vi "Draw Flattened Pixmap.vi"(8 "image data":T1, 9 "picture":picture) -> (3 "new picture":picture)   [LabVIEW 2011]
doc: "Draws a 1-, 4-, or 8-bit pixmap or a 24-bit RGB pixmap into a picture."
uses:
  imagedata.ctl
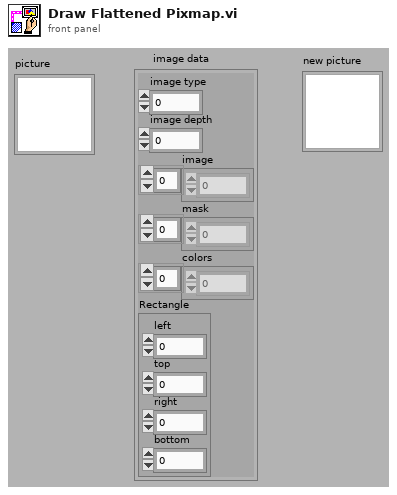
[diagram p1: front panel]
types:
  T1 = typedef "imagedata.ctl" = cluster{"image type":i32, "image depth":i32, "image":u8[], "mask":u8[], "colors":u32[], "Rectangle":cluster{"left":i16, "top":i16, "right":i16, "bottom":i16}}
  T2 = cluster{"left":i16, "top":i16, "right":i16, "bottom":i16}
  T3 = cluster{"top":i16, "left":i16, "bottom":i16, "right":i16}
  T4 = cluster{"default foreground":u32, "default background":u32}
  T5 = cluster{"opcode-Copy Pixmap":i16, i32, i32, cluster{"top":i16, "left":i16, "bottom":i16, "right":i16}, i16, cluster{"default foreground":u32, "default background":u32}}
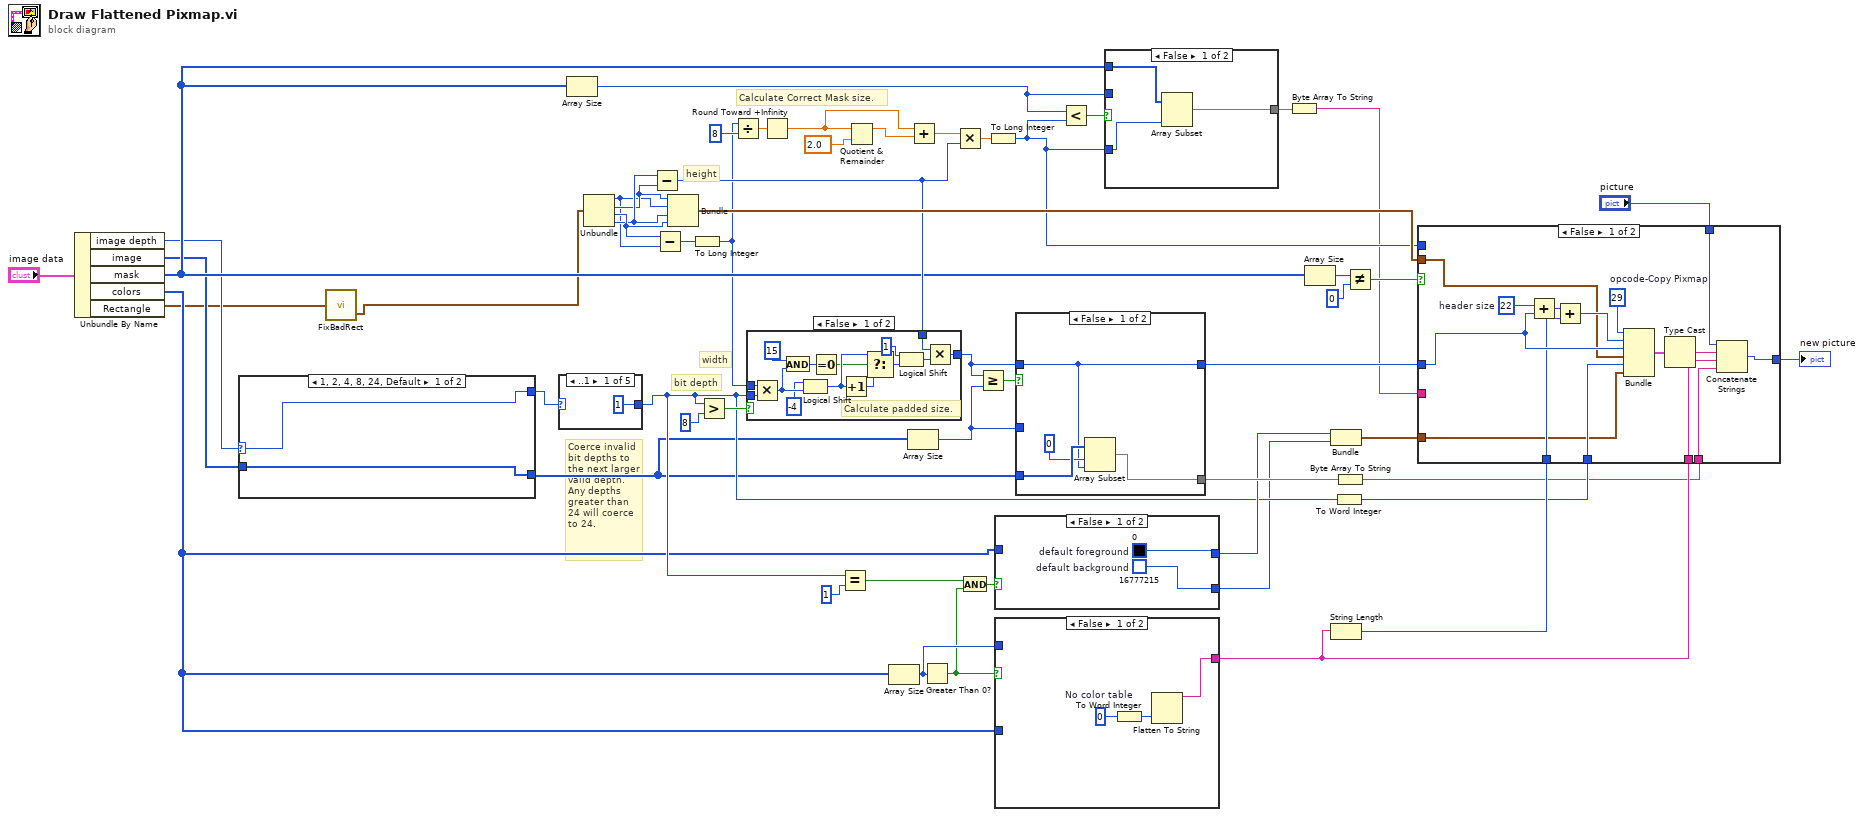
[diagram p0: block diagram]
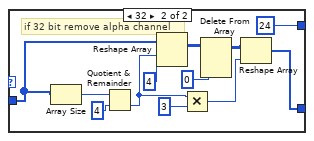
[diagram p2: hidden frame]
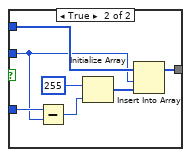
[diagram p3: hidden frame]
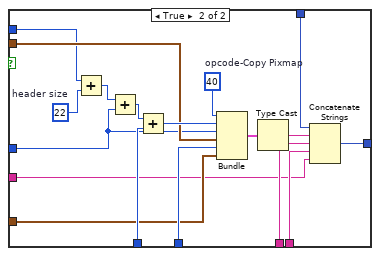
[diagram p4: hidden frame]
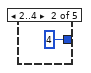
[diagram p5: hidden frame]
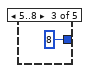
[diagram p6: hidden frame]
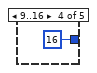
[diagram p7: hidden frame]
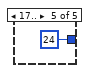
[diagram p8: hidden frame]
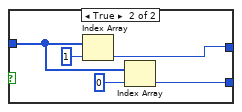
[diagram p9: hidden frame]
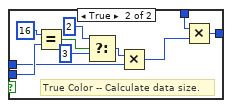
[diagram p10: hidden frame]
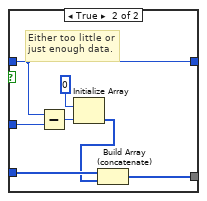
[diagram p11: hidden frame]
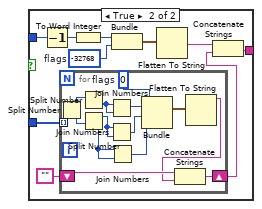
[diagram p12: hidden frame]
diagram:
  # "Calculate Correct Mask size."
  # "Coerce invalid\nbit depths to\nthe next larger\nvalid depth.\nAny depths\ngreater than\n24 will coerce\nto 24."
  # "bit depth"
  # "height"
  # "width"
  n1 = Unbundle By Name("image data") -> ("image depth"=w6:i32, "image"=w5:u8[], "mask"=w11:u8[], "colors"=w18:u32[], "Rectangle"=w2:T2)
  n2 = case shown="1, 2, 4, 8, 24, Default" w6 {
    selector: w6 -> [w56 _]
    tunnel: [w56 24] -> w3
    tunnel: w5 -> [w55 w67]
    tunnel: [w55 w58] -> w4
    frame 1, 2, 4, 8, 24, Default {
    }
    frame 32 {
      # "if 32 bit remove alpha channel"
      n3 = Array Size(array=w67) -> (size(s)=w66:i32)
      n4 = Quotient & Remainder(x=w66, y=4) -> (floor(x/y)=w62:i32)  [unwired: 1 out]
      n5 = Reshape Array(w67, w62, 4 ("dimension size")) -> (w64:u8[][])
      n6 = Multiply(x=w62, y=3) -> (x*y=w60:i32)
      n7 = Delete From Array(array=w64, index (col)=0 ("dimension size")) -> (array with subset deleted=w59:u8[][])  [unwired: 2 in, 1 out]
      n8 = Reshape Array(w59, w60) -> (w58:u8[])
    }
  }
  n9 = call "FixBadRect.vi"("Rectangle In"=w2) -> ("Rectangle Out"=w1:T2)  [unwired: 1 out]
  n10 = case shown="..1" w3 {
    tunnel: [1 4 8 16 24] -> w33
    frame ..1 {
    }
    frame 2..4 {
    }
    frame 5..8 {
    }
    frame 9..16 {
    }
    frame 17.. {
    }
  }
  n11 = Array Size(array=w11) -> (size(s)=w13:i32)
  n12 = Unbundle(w1) -> ("left"=w8:i16, "top"=w46:i16, "right"=w48:i16, "bottom"=w47:i16)
  n13 = Subtract(x=w47, y=w46) -> (x-y=w15:i16)
  n14 = Subtract(x=w48, y=w8) -> (x-y=w22:i16)
  n15 = Bundle("top"=w46, "left"=w8, "bottom"=w47, "right"=w48) -> (w17:T3)  [unwired: 1 out]
  n16 = To Long Integer(number=w22) -> (32bit integer=w7:i32)
  n17 = Greater?(x=w33, y=u8 8) -> (0:w39:bool)
  n18 = Divide(x=w7, y=8) -> (x/y=w27:dbl)
  n19 = case shown="False" w39 {
    tunnel: [w87 w97] -> w44
    tunnel: w15 -> [w83 w96]
    tunnel: w33 -> [w75 w94]
    tunnel: w7 -> [w74 w92]
    frame False {
      # "Calculate padded size."
      n20 = Multiply(x=w74, y=w75) -> (x*y=w77:i32)
      n21 = And(x=15, y=w77) -> (x .and. y?=w79:i32)
      n22 = Logical Shift(y=-4, x=w77) -> (x << y=w81:i32)
      n23 = Equal To 0?(x=w79) -> (x = 0?=w80:bool)
      n24 = Increment(x=w81) -> (x+1=w82:i32)
      n25 = Select(t=w81, s=w80, f=w82) -> (s? t:f=w85:i32)
      n26 = Logical Shift(y=1, x=w85) -> (x << y=w86:i32)
      n27 = Multiply(x=w83, y=w86) -> (x*y=w87:i32)
    }
    frame True {
      # "True Color -- Calculate data size."
      n28 = Equal?(x=16, y=w94) -> (x = y?=w91:bool)
      n29 = Select(t=2, s=w91, f=3) -> (s? t:f=w88:i32)
      n30 = Multiply(x=w88, y=w92) -> (x*y=w95:i32)
      n31 = Multiply(x=w96, y=w95) -> (x*y=w97:i32)
    }
  }
  n32 = Round Toward +Infinity(x=w27) -> (ceil(x): smallest int >= x=w26:dbl)
  n33 = Equal?(x=w33, y=u8 1) -> (x = y?=w34:bool)
  n34 = Quotient & Remainder(x=w26, y=2.0) -> (x-y*floor(x/y)=w31:dbl)  [unwired: 1 out]
  n35 = Array Size(array=w18) -> (size(s)=w54:i32)
  n36 = Array Size(array=w4) -> (size(s)=w42:i32)
  n37 = Add(x=w26, y=w31) -> (x+y=w16:dbl)
  n38 = Greater Than 0?(x=w54) -> (x > 0?=w36:bool)
  n39 = Multiply(x=w16, y=w15) -> (x*y=w30:dbl)
  n40 = And(x=w34, y=w36) -> (x .and. y?=w37:bool)
  n41 = Greater Or Equal?(x=w44, y=w42) -> (x >= y?=w45:bool)
  n42 = To Long Integer(number=w30) -> (32bit integer=w12:i32)
  n43 = case shown="False" w37 {
    tunnel: [w99 w100] -> w38
    tunnel: [w98 w101] -> w24
    tunnel: w18 -> [_ w102]
    frame False {
      w98 = u32 16777215  # default background
      w99 = u32 0  # default foreground
    }
    frame True {
      n44 = Index Array(array=w102, index=1) -> (element=w100:u32)
      n45 = Index Array(array=w102, index=0) -> (element=w101:u32)
    }
  }
  n46 = case shown="False" w36 {
    tunnel: w18 -> [_ w108]
    tunnel: w54 -> [_ w117]
    tunnel: [w105 w112] -> w51
    frame False {
      w107 = 0  # No color table
      n47 = To Word Integer(number=w107) -> (16bit integer=w106:i16)
      n48 = Flatten To String(anything=w106) -> (data string=w105:string)  [unwired: 1 in, 4 out]
    }
    frame True {
      w115 = i16 -32768  # flags
      n49 = Decrement(x=w117) -> (x-1=w109:i32)
      n50 = for {
        tunnel: w108 -> [w129] mode=indexing
        shift-right: [w126] -> w110
        shift-left: "" -> [w127]
        w128 = i16 0  # flags
        n51 = Split Number(x=w129) -> (hi(x)=w131:u16, lo(x)=w130:u16)
        n52 = Split Number(x=w131) -> (lo(x)=w118:u8)  [unwired: 1 out]
        n53 = Split Number(x=w130) -> (hi(x)=w124:u8, lo(x)=w123:u8)
        n54 = Join Numbers(hi=w118, lo=w118) -> ((hi.lo)=w125:u16)
        n55 = Join Numbers(hi=w124, lo=w124) -> ((hi.lo)=w122:u16)
        n56 = Join Numbers(hi=w123, lo=w123) -> ((hi.lo)=w121:u16)
        n57 = Bundle("flags"=w128, w125, w122, w121) -> (w120:cluster{"flags":i16, u16, u16, u16})  [unwired: 1 out]
        n58 = Flatten To String(anything=w120) -> (data string=w119:string)  [unwired: 1 in, 4 out]
        n59 = Concatenate Strings(w127, w119) -> (w126:string)
      }
      n60 = To Word Integer(number=w109) -> (16bit integer=w116:i16)
      n61 = Bundle(w116, "flags"=w115) -> (w114:cluster{i16, "flags":i16})  [unwired: 1 out]
      n62 = Flatten To String(anything=w114) -> (data string=w113:string)  [unwired: 1 in, 4 out]
      n63 = Concatenate Strings(w113, w110) -> (w112:string)
    }
  }
  n64 = case shown="False" w45 {
    tunnel: w4 -> [w135 w139]
    tunnel: [w134 w140] -> w41
    tunnel: w44 -> [w132 w136]
    tunnel: [w132 w136] -> w43
    tunnel: w42 -> [_ w137]
    frame False {
      n65 = Array Subset(array=w135, index=0, length=w132) -> (w134:u8[])
    }
    frame True {
      # "Either too little or\njust enough data."
      n66 = Subtract(x=w136, y=w137) -> (x-y=w142:i32)
      n67 = Initialize Array(u8 0, w142) -> (w138:u8[])
      n68 = Build Array (concatenate)(w139, w138) -> (w140:u8[])
    }
  }
  n69 = Less?(x=w13, y=w12) -> (x < y?=w14:bool)
  n70 = case shown="False" w14 {
    tunnel: w11 -> [w145 w148]
    tunnel: w13 -> [_ w147]
    tunnel: w12 -> [w144 w151]
    tunnel: [w143 w146] -> w10
    frame False {
      n71 = Array Subset(array=w145, length=w144) -> (w143:u8[])  [unwired: 1 in]
    }
    frame True {
      n72 = Subtract(x=w151, y=w147) -> (x-y=w150:i32)
      n73 = Initialize Array(u8 255 ("element"), w150) -> (w149:u8[])
      n74 = Insert Into Array(array=w148, index=w147, new element=w149) -> (w146:u8[])
    }
  }
  n75 = Byte Array To String(unsigned byte array=w10) -> (string=w9:string)
  n76 = Array Size(array=w11) -> (size(s)=w23:i32)
  n77 = Bundle("default foreground"=w38, "default background"=w24) -> (w49:T4)  [unwired: 1 out]
  n78 = String Length(string=w51) -> (length=w53:i32)
  n79 = To Word Integer(number=w33) -> (16bit integer=w52:i16)
  n80 = Byte Array To String(unsigned byte array=w41) -> (string=w50:string)
  n81 = Not Equal?(x=w23, y=0) -> (x != y?=w29:bool)
  n82 = case shown="False" w29 {
    tunnel: w53 -> [w158 w182]
    tunnel: w52 -> [w157 w180]
    tunnel: [w153 w179] -> w21
    tunnel: w51 -> [w160 w178]
    tunnel: w50 -> [w159 w177]
    tunnel: w49 -> [w156 w175]
    tunnel: w17 -> [w155 w174]
    tunnel: w43 -> [w161 w173]
    tunnel: w12 -> [_ w172]
    tunnel: w9 -> [_ w168]
    tunnel: "picture" -> [w154 w169]
    frame False {
      w164 = i16 22  # header size
      w162 = i16 29  # opcode-Copy Pixmap
      n83 = Add(x=w164, y=w161) -> (x+y=w165:i32)
      n84 = Add(x=w165, y=w158) -> (x+y=w166:i32)
      n85 = Bundle("opcode-Copy Pixmap"=w162, w166, w161, w155, w157, w156) -> (w163:T5)  [unwired: 1 out]
      n86 = Type Cast(x=w163) -> (*(type *) &x=w167:string)  [unwired: 1 out]
      n87 = Concatenate Strings(w154, w167, w160, w159) -> (w153:picture)
    }
    frame True {
      w185 = i16 40  # opcode-Copy Pixmap
      w170 = i16 22  # header size
      n88 = Add(x=w172, y=w170) -> (x+y=w171:i32)
      n89 = Add(x=w171, y=w173) -> (x+y=w183:i32)
      n90 = Add(x=w183, y=w182) -> (x+y=w181:i32)
      n91 = Bundle("opcode-Copy Pixmap"=w185, w181, w173, w174, w180, w175) -> (w184:T5)  [unwired: 1 out]
      n92 = Type Cast(x=w184) -> (*(type *) &x=w176:string)  [unwired: 1 out]
      n93 = Concatenate Strings(w169, w176, w178, w177, w168) -> (w179:picture)
    }
  }
  "new picture" <- w21
